vi "GetBounds.vi"(0 "XRef":T5, 1 "State In":T4) -> (14 "Bounds":T2, 15 "Fatal Error Out":T1)   [LabVIEW 2015, in "LVJSON.lvlib" / "Build JSON Array.xnode"]
uses:
  Build JSON Array.xnode
  <vilib>/XNodeSupport/XNodeXNodeRef.ctl
  State.ctl
  <vilib>/XNodeSupport/XNodeBounds.ctl
  <vilib>/XNodeSupport/XNodeInt.ctl
  <vilib>/XNodeSupport/XNodeErrorCluster.ctl
  dimensions.vi
  <vilib>/XNodeSupport/NI_XNodeSupport.lvlib
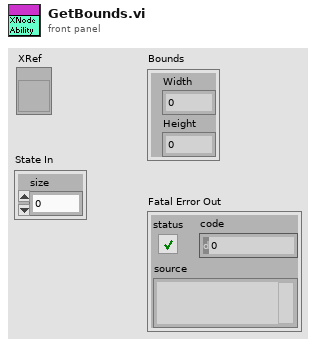
[diagram p1: front panel]
types:
  T1 = typedef "NI_XNodeSupport.lvlib/XNodeErrorCluster.ctl" = errorcluster
  T2 = typedef "NI_XNodeSupport.lvlib/XNodeBounds.ctl" = cluster{"Width":T3, "Height":T3}
  T3 = typedef "NI_XNodeSupport.lvlib/XNodeInt.ctl" = i32
  T4 = typedef "LVJSON.lvlib/Build JSON Array.xnode/State.ctl" = cluster{"size":u32}
  T5 = typedef "NI_XNodeSupport.lvlib/XNodeXNodeRef.ctl" = refnum<vi>
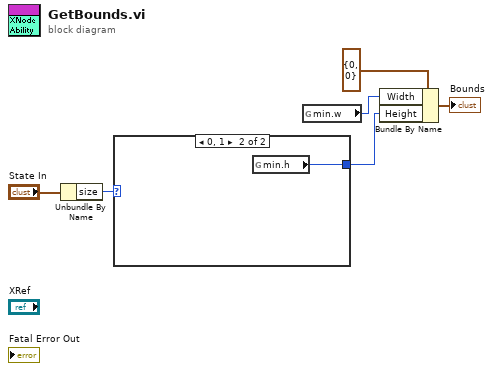
[diagram p0: block diagram]
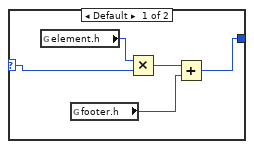
[diagram p2: hidden frame]
diagram:
  n1 = Unbundle By Name("State In") -> ("size"=w5:u32)
  n2 = case shown="0, 1" w5 {
    selector: w5 -> [w10 _]
    tunnel: [w11 w12] -> w2
    frame Default {
      n3 = global read "dimensions.vi" "element.h"() -> (w9:i16)
      n4 = global read "dimensions.vi" "footer.h"() -> (w7:i16)
      n5 = Multiply(x=w9, y=w10) -> (x*y=w8:u32)
      n6 = Add(x=w8, y=w7) -> (x+y=w11:u32)
    }
    frame 0, 1 {
      n7 = global read "dimensions.vi" "min.h"() -> (w12:i32)
    }
  }
  n8 = global read "dimensions.vi" "min.w"() -> (w3:i32)
  n9 = Bundle By Name(cluster=T2 {"Width"=0, "Height"=0} ("Bounds"), "Width"=w3, "Height"=w2) -> (→"Bounds":T2)
